vi "U3 DAC_global_save.vi"() -> ()   [LabVIEW 2016]
panel:
  in  "Numeric":dbl
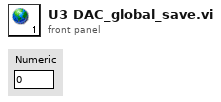
[diagram p1: front panel]
diagram:
